vi "Process CDIR.vi"(11 "FHPP in":refnum<class "FHPP.lvclass">) -> (3 "FHPP out":refnum<class "FHPP.lvclass">)   [LabVIEW 2022 SP3, in "FHPP.lvclass"]
uses:
  FHPP.lvclass
  FHPP.lvclass/FHPP.ctl
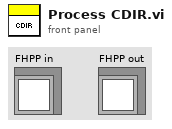
[diagram p1: front panel]
types:
  T1 = typedef "FHPP.lvclass/DIR.ctl" = cluster{"Relative":bool, "Control Mode":enum8{"Position", "Force", "Velocity", "Reserved"}, "Function":enum8{"Reserved", "External Input", "External Input with  Cam", "Virtual Master with Cam"}, "Function Group":enum8{"No Function", "Reserver 1", "Reserved 2", "Reserved 3"}, "Camming":bool}
  T2 = typedef "FHPP.lvclass/Setpoints.ctl" = cluster{"Vel/VelRamp (%)":u8, "Setpoint":u32}
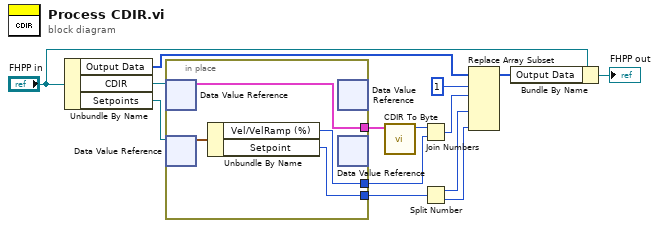
[diagram p0: block diagram]
diagram:
  n1 = Unbundle By Name("FHPP in") -> ("Output Data"=w10:u16[], "CDIR"=w9:refnum<data-value>, "Setpoints"=w5:refnum<data-value>)
  n2 = in-place {
    in-place-border: [w18] -> w7
    in-place-border: [w16] -> w4
    in-place-border: [w15] -> w3
    n3 = in-place-dvr #1(w9) -> (w18:T1)  [unwired: 1 out]
    n4 = in-place-dvr #2(w5) -> (w17:T2)  [unwired: 1 out]
    n5 = Unbundle By Name(w17) -> ("Vel/VelRamp (%)"=w16:u8, "Setpoint"=w15:u32)
    n6 = in-place-dvr #1() -> ()  [unwired: 1 in, 2 out]
    n7 = in-place-dvr #2() -> ()  [unwired: 1 in, 2 out]
  }
  n8 = call "CDIR To Byte.vi"("DIR"=w7) -> ("Numeric"=w6:u8)  [unwired: 10 in]
  n9 = Join Numbers(hi=w6, lo=w4) -> ((hi.lo)=w12:u16)
  n10 = Split Number(x=w3) -> (hi(x)=w2:u16, lo(x)=w1:u16)
  n11 = Replace Array Subset(array=w10, new element #1=w12, index #1=1 ("index"), new element #2=w2, new element #3=w1) -> (w13:u16[])  [unwired: 2 in]
  n12 = Bundle By Name(cluster="FHPP in", "Output Data"=w13) -> (→"FHPP out":refnum<class "FHPP.lvclass">)
